vi "DataLog Append String.vi"(0 "tag log directory":path, 7 "string":string, 11 "error in (no error)":errorcluster) -> (4 "dup tag log directory":path, 6 "offset":dbl, 8 "dup string":string, 15 "error out":errorcluster)   [LabVIEW 2012]
doc: "Append a string to the strings file in a string tag's log directory. Returns the offset at which the string was written."
uses:
  glb_DataLog MCVD.vi
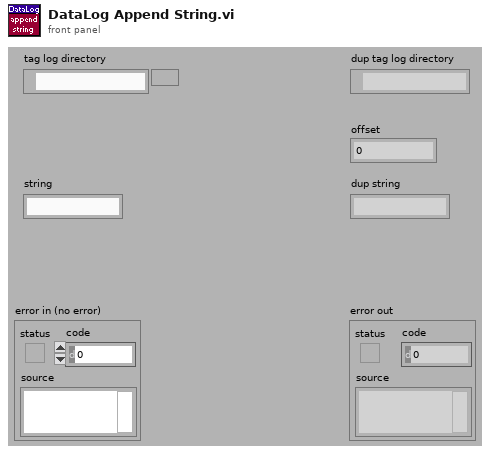
[diagram p1: front panel]
types:
  T1 = enum16{"deny read/write", "deny write-only", "deny none"}
  T2 = enum16{"read/write", "read-only", "write-only", "write-only (truncate)"}
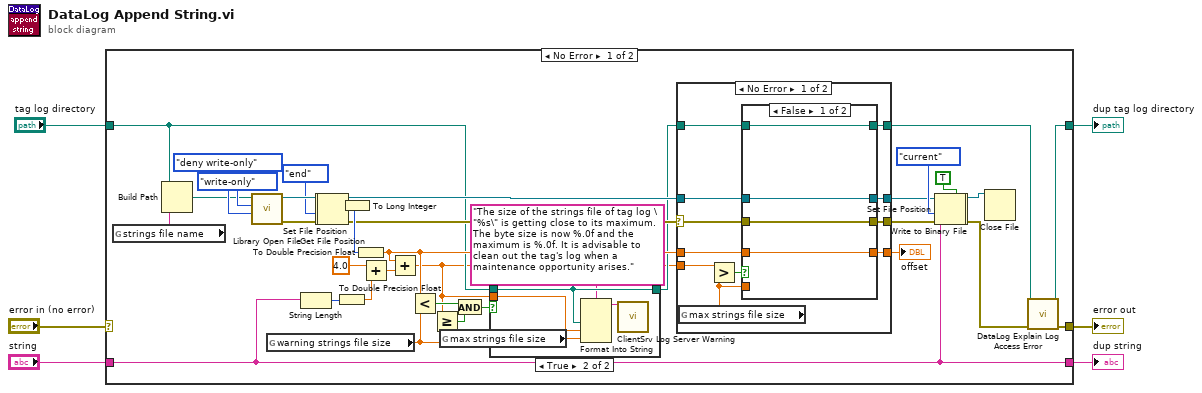
[diagram p0: block diagram]
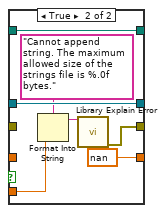
[diagram p3: hidden frame]
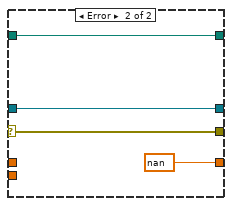
[diagram p4: hidden frame]
diagram:
  n1 = case shown="No Error" "error in (no error)" {
    selector: "error in (no error)" -> [_ w79]
    tunnel: [w25 w79] -> w6
    tunnel: "tag log directory" -> [w15 w78]
    tunnel: [w22 w78] -> w3
    tunnel: "string" -> [w21 w77]
    tunnel: [w21 w77] -> w1
    frame No Error {
      n2 = global read "glb_DataLog MCVD.vi" "strings file name"() -> (w42:string)
      n3 = Build Path(base path=w15, name or relative path=w42) -> (appended path=w41:path)
      n4 = call "Library Open File.vi"("deny mode (deny none)"=T1."deny write-only" ("deny mode (2)"), "open mode (read/write)"=T2."write-only" ("open mode (0)"), "file path"=w41) -> ("error out"=w40:errorcluster, "refnum"=w39:refnum<file>)  [unwired: 3 in]
      n5 = global read "glb_DataLog MCVD.vi" "warning strings file size"() -> (w16:dbl)
      n6 = String Length(string=w21) -> (length=w35:i32)
      n7 = Set File Position(refnum=w39, from (0:start)=enum16{"start", "end", "current"}."end" ("pos mode (0:2)"), error in=w40) -> (refnum out=w9:refnum<file>, error out=w8:errorcluster)  [unwired: 1 in]
      n8 = Get File Position(4:w8, 7:w9) -> (0:w33:errorcluster, 2:w7:i64, 3:w30:refnum<file>)
      n9 = To Double Precision Float(number=w35) -> (double precision float=w27:dbl)
      n10 = To Long Integer(number=w7) -> (32bit integer=w37:i32)
      n11 = To Double Precision Float(number=w37) -> (double precision float=w18:dbl)
      n12 = Add(x=4.0, y=w27) -> (x+y=w28:dbl)
      n13 = Add(x=w18, y=w28) -> (x+y=w13:dbl)
      n14 = Less?(x=w18, y=w16) -> (x < y?=w20:bool)
      n15 = Greater Or Equal?(x=w13, y=w16) -> (x >= y?=w19:bool)
      n16 = And(x=w20, y=w19) -> (x .and. y?=w17:bool)
      n17 = case shown="True" w17 {
        tunnel: w15 -> [w45 w50]
        tunnel: [w45 w50] -> w14
        tunnel: w13 -> [_ w47]
        frame False {
        }
        frame True {
          n18 = global read "glb_DataLog MCVD.vi" "max strings file size"() -> (w46:dbl)
          n19 = Format Into String(format string="The size of the strings file of tag log \"%s\" is getting close to its maximum. The byte size is now %.0f and the maximum is %.0f. It is advisable to clean out the tag's log when a maintenance opportunity arises.", w50, w47, w46) -> (resulting string=w49:string)  [unwired: 2 in, 1 out]
          n20 = call "ClientSrv Log Server Warning.vi"("message (use cluster)"=w49) -> ()  [unwired: 15 in]
        }
      }
      n21 = case shown="No Error" w33 {
        selector: w33 -> [w61 w76]
        tunnel: [w60 w76] -> w34
        tunnel: w14 -> [w58 w75]
        tunnel: [w57 w75] -> w23
        tunnel: w13 -> [w53 _]
        tunnel: [w56 nan ("x+y")] -> w31
        tunnel: w30 -> [w55 w73]
        tunnel: [w54 w73] -> w29
        tunnel: w18 -> [w52 _]
        frame No Error {
          n22 = global read "glb_DataLog MCVD.vi" "max strings file size"() -> (w51:dbl)
          n23 = Greater?(x=w53, y=w51) -> (0:w59:bool)
          n24 = case shown="False" w59 {
            tunnel: w61 -> [w62 _]
            tunnel: [w62 w72] -> w60
            tunnel: w58 -> [w65 w67]
            tunnel: [w65 w67] -> w57
            tunnel: [w64 nan ("x+y")] -> w56
            tunnel: w52 -> [w64 _]
            tunnel: [w63 w70] -> w54
            tunnel: w55 -> [w63 w70]
            tunnel: w51 -> [_ w68]
            frame False {
            }
            frame True {
              n25 = Format Into String(format string="Cannot append string. The maximum allowed size of the strings file is %.0f bytes.", w68) -> (resulting string=w69:string)  [unwired: 2 in, 1 out]
              n26 = call "Library Explain Error.vi"("explanation prefix (none)"=w69) -> ("explained error"=w72:errorcluster)  [unwired: 14 in]
            }
          }
        }
        frame Error {
        }
      }
      "offset" <- w31
      n27 = Set File Position(refnum=w29, from (0:start)=enum16{"start", "end", "current"}."current" ("pos mode (0:2)"), error in=w34) -> (refnum out=w11:refnum<file>, error out=w10:errorcluster)  [unwired: 1 in]
      n28 = Write to Binary File(file (use dialog)=w11, data=w21, error in=w10, 5:TRUE ("header (F)")) -> (refnum out=w32:refnum<file>, error out=w24:errorcluster)  [unwired: 2 in, 1 out]
      n29 = Close File(refnum=w32) -> ()  [unwired: 1 in, 2 out]
      n30 = call "DataLog Explain Log Access Error.vi"("tag log directory"=w23, "error in"=w24) -> ("dup tag log directory"=w22:path, "error out"=w25:errorcluster)  [unwired: 12 in]
    }
    frame Error {
    }
  }
  "error out" <- w6
  "dup tag log directory" <- w3
  "dup string" <- w1
